vi "Visible (SubVI).vi"(1 "relatCoord":cluster{"x relat ":i32, "y relat":i32}) -> (0 "output cluster":T1)   [LabVIEW 2011]
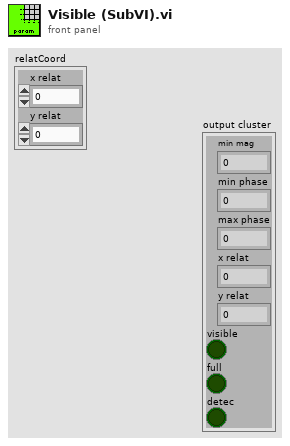
[diagram p1: front panel]
types:
  T1 = cluster{"min mag":dbl, "min phase":dbl, "max phase":dbl, "x relat":i32, "y relat":i32, "visible":bool, "full":bool, "detec":bool}
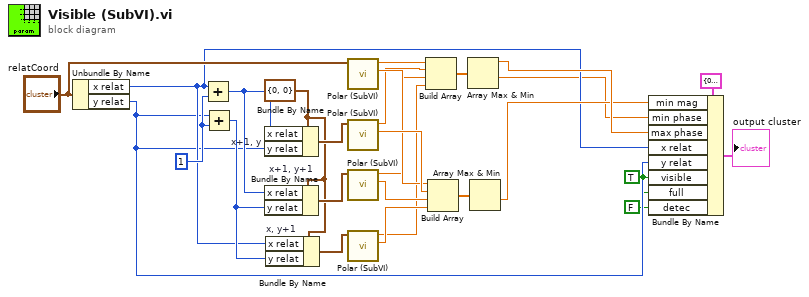
[diagram p0: block diagram]
diagram:
  w7 = 1 ("cell")
  w3 = TRUE ("visible")
  w9 = cluster{"x relat":i32, "y relat":i32} {"x relat"=0, "y relat"=0} ("input cluster")
  n1 = Unbundle By Name("relatCoord") -> ("x relat"=w6:i32, "y relat"=w5:i32)
  n2 = Add(x=w6, y=w7) -> (x+y=w10:i32)
  n3 = Add(x=w5, y=w7) -> (x+y=w11:i32)
  n4 = Bundle By Name "x+1, y"(cluster=w9, "x relat"=w10, "y relat"=w5) -> (w12:cluster{"x relat":i32, "y relat":i32})
  n5 = Bundle By Name "x+1, y+1"(cluster=w9, "x relat"=w10, "y relat"=w11) -> (w13:cluster{"x relat":i32, "y relat":i32})
  n6 = Bundle By Name "x, y+1"(cluster=w9, "x relat"=w6, "y relat"=w11) -> (w14:cluster{"x relat":i32, "y relat":i32})
  n7 = call "Polar (SubVI).vi"("priorCoord"="relatCoord") -> ("magnitude"=w20:dbl, "phase"=w15:dbl)  [unwired: 9 in]
  n8 = call "Polar (SubVI).vi"("priorCoord"=w12) -> ("magnitude"=w21:dbl, "phase"=w16:dbl)  [unwired: 9 in]
  n9 = call "Polar (SubVI).vi"("priorCoord"=w13) -> ("magnitude"=w22:dbl, "phase"=w17:dbl)  [unwired: 9 in]
  n10 = call "Polar (SubVI).vi"("priorCoord"=w14) -> ("magnitude"=w23:dbl, "phase"=w18:dbl)  [unwired: 9 in]
  n11 = Build Array(w15, w16, w17, w18) -> (w19:dbl[])
  n12 = Build Array(w20, w21, w22, w23) -> (w24:dbl[])
  n13 = Array Max & Min(array=w19) -> (max value=w26:dbl, min value=w4:dbl)  [unwired: 2 out]
  n14 = Array Max & Min(array=w24) -> (min value=w25:dbl)  [unwired: 3 out]
  n15 = Bundle By Name(cluster=T1 {"min mag"=0.0, "min phase"=0.0, "max phase"=0.0, "x relat"=0, "y relat"=0, "visible"=TRUE, "full"=TRUE, "detec"=TRUE} ("input cluster"), "min mag"=w25, "min phase"=w4, "max phase"=w26, "x relat"=w6, "y relat"=w5, "visible"=w3, "full"=w3, "detec"=FALSE) -> (→"output cluster":T1)
